vi "PWM.vi"() -> ()   [LabVIEW 2020]
uses:
  <vilib>/MakerHub/LINX/Public/Utilities/Open Serial.vi
  <vilib>/MakerHub/LINX/Public/Peripherals/PWM/PWM Set Duty Cycle N Chans.vi
  <vilib>/MakerHub/LINX/LMH-LINX.lvlib
panel:
  in  "Blue Phase":dbl(knob) caption="Phase" min=0.0 max=360.0 scale=0.0..360.0
  in  "Green Phase":dbl(knob) caption="Phase" min=0.0 max=360.0 scale=0.0..360.0
  out "RGB LED Color":u32(colorbox)
  in  "Red Amplitude":dbl(slide)=0.5 caption="Amplitude" min=0.0 max=0.5 step=0.01 scale=0.0..0.5
  in  "Blue Amplitude":dbl(slide)=0.5 caption="Amplitude" min=0.0 max=0.5 step=0.01 scale=0.0..0.5
  in  "Green Amplitude":dbl(slide)=0.5 caption="Amplitude" min=0.0 max=0.5 step=0.01 scale=0.0..0.5
  in  "Red Phase":dbl(knob) caption="Phase" min=0.0 max=360.0 scale=0.0..360.0
  in  "Frequency":dbl(slide)=1.0 scale=0.0..1.0
  in  "Stop Button":bool
  in  "Channels":u8[](array[numeric]) min=9 max=9
  in  "Serial Port":refnum<visa-resource-name>="N/A"
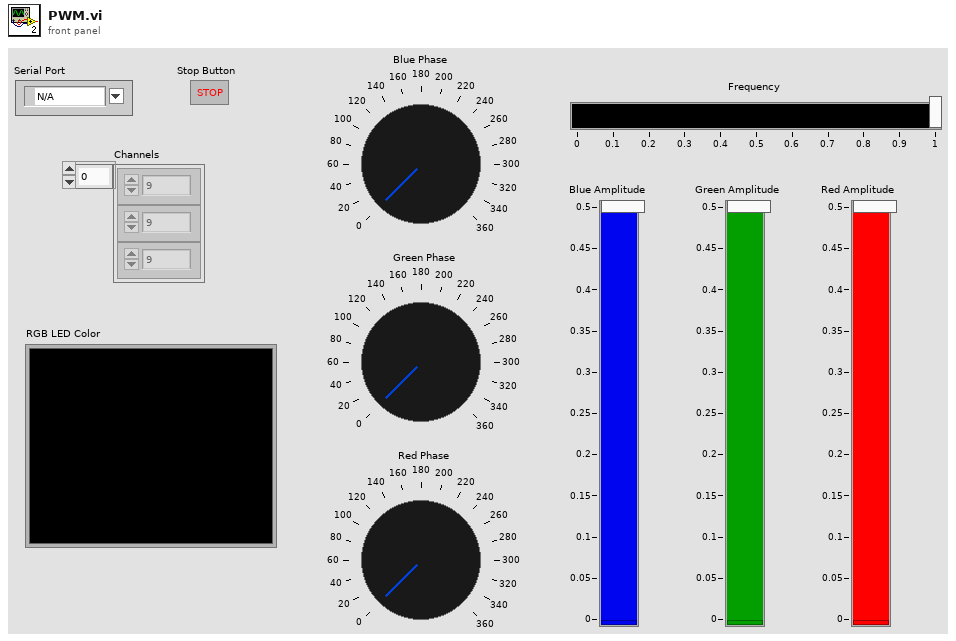
[diagram p1: front panel]
types:
  T1 = typedef "LMH-LINX.lvlib/LINX Ref.ctl" = cluster{"IO":T2, "Interface":T3, "LINX Device Config":T4}
  T2 = typedef "LMH-LINX.lvlib/Platform.ctl" = enum16{"Remote", "Local"}
  T3 = typedef "LMH-LINX.lvlib/Interface.ctl" = enum16{"Serial", "TCP"}
  T4 = typedef "LMH-LINX.lvlib/Device.lvlib/LINX Device Config.ctl" = cluster{"Interface":T3, "COM Port":refnum<visa-resource-name>, "TCP Configuration":T5, "Device Family":u8, "Device ID":u8, "Device Name":string, "TCP Ref":refnum<k5>, "Channels":T6}
  T5 = typedef "LMH-LINX.lvlib/Device.lvlib/TCP Config.ctl" = cluster{"IP Address":string, "Port":u16}
  T6 = typedef "LMH-LINX.lvlib/Channels.ctl" = cluster{"DI":u8[], "DO":u8[], "AI":u8[], "AO":u8[], "PWM":u8[], "QE":u8[], "UART":u8[], "I2C 2":u8[], "SPI":u8[], "CAN":u8[], "Servo":u8[], "AI Ref (V)":dbl, "AI Resolution (Bits)":u8, "AO Ref (V)":dbl, "AO Resolution (Bits)":u8}
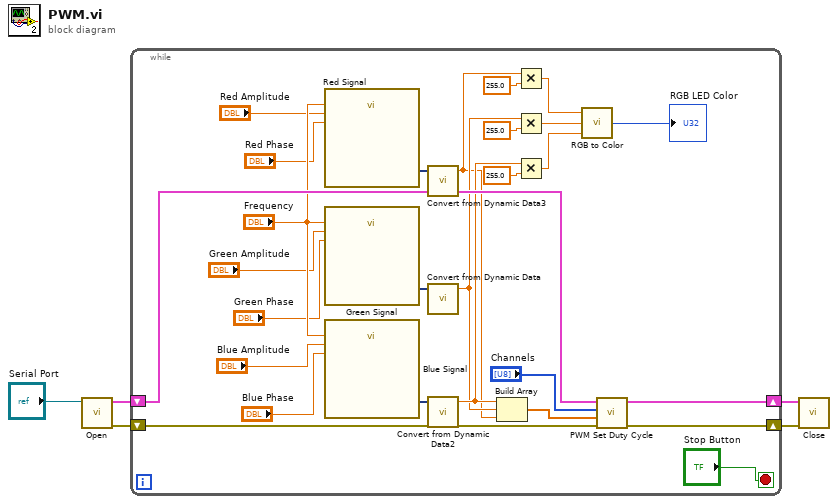
[diagram p0: block diagram]
diagram:
  n1 = call-poly <vilib>:"Open.vi"("Serial Port"="Serial Port") -> ("Error Out"=w2:errorcluster, "LINX Resource"=w4:T1)  [unwired: 8 in, 1 out]
  n2 = while {
    shift-right: [w31] -> w3
    shift-left: w4 -> [w32]
    shift-right: [w29] -> w1
    shift-left: w2 -> [w30]
    stop <- "Stop Button" stop-if-true
    n3 = call "Red Signal"("Frequency"="Frequency", "Amplitude"="Red Amplitude", "Phase"="Red Phase") -> ("Sine"=w21:dynamicdata)  [unwired: 11 in, 1 out]
    n4 = call "Green Signal"("Frequency"="Frequency", "Amplitude"="Green Amplitude", "Phase"="Green Phase") -> ("Sine"=w23:dynamicdata)  [unwired: 11 in, 1 out]
    n5 = call "Blue Signal"("Frequency"="Frequency", "Amplitude"="Blue Amplitude", "Phase"="Blue Phase") -> ("Sine"=w22:dynamicdata)  [unwired: 11 in, 1 out]
    n6 = call "Convert from Dynamic Data3"("Dynamic Data Type"=w21) -> ("Scalar"=w12:dbl)  [unwired: 3 in]
    n7 = call "Convert from Dynamic Data"("Dynamic Data Type"=w23) -> ("Scalar"=w13:dbl)  [unwired: 3 in]
    n8 = call "Convert from Dynamic Data2"("Dynamic Data Type"=w22) -> ("Scalar"=w14:dbl)  [unwired: 3 in]
    n9 = Build Array(w14, w13, w12) -> (w27:dbl[])
    n10 = Multiply(x=w12, y=255.0) -> (x*y=w17:dbl)
    n11 = Multiply(x=w13, y=255.0) -> (x*y=w16:dbl)
    n12 = Multiply(x=w14, y=255.0) -> (x*y=w15:dbl)
    n13 = call <vilib>:"RGB to Color.vi"("B"=w15, "G"=w16, "R"=w17) -> ("Color"=→"RGB LED Color":u32)
    n14 = call-poly <vilib>:"PWM Set Duty Cycle.vi"("Error In"=w30, "Duty Cycles"=w27, "PWM Channels"="Channels", "LINX Resource"=w32) -> ("Error Out"=w29:errorcluster, "LINX Resource"=w31:T1)  [unwired: 6 in]
  }
  n15 = call <vilib>:"Close.vi"("Error In"=w1, "LINX Resource"=w3) -> ()  [unwired: 9 in, 1 out]
